vi "1基礎題-Enum-combo box.vi"() -> ()   [LabVIEW 2019]
panel:
  in  "Stop":bool
  out "結果":string
  in  "板材":enum16{"¬üªäªO", "§¨ªO"}(ring)
  in  "色號":string(combo)="フ撤━"
  # "選擇不同的板材時，會出現對應的色號選項供使用者選擇\n並在結果顯示使用者選擇的結果"
  # "Enum"
  # "Combo Box"
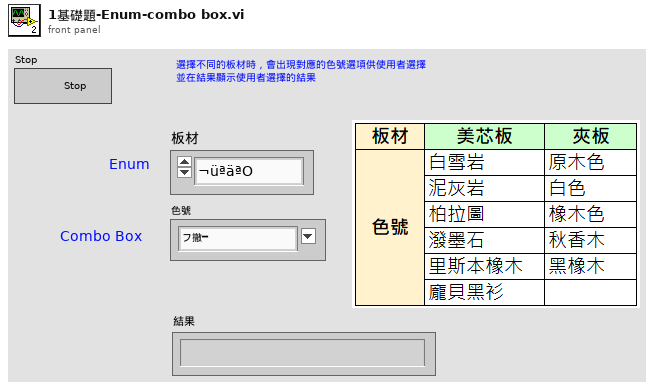
[diagram p1: front panel]
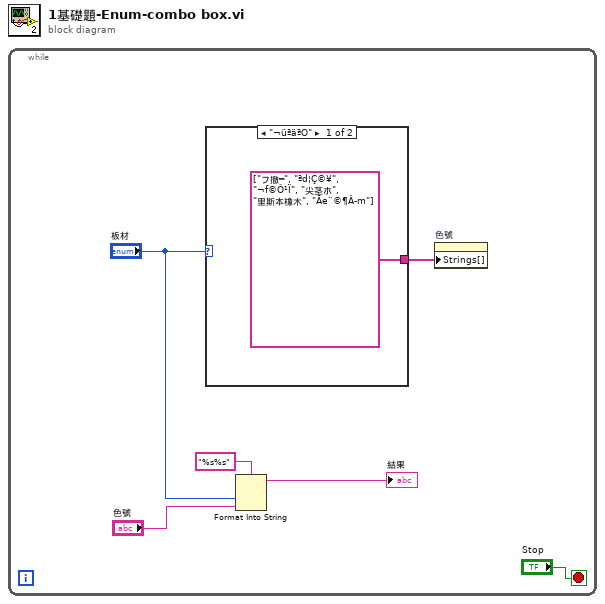
[diagram p0: block diagram]
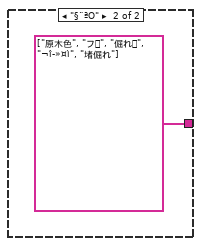
[diagram p2: hidden frame]
diagram:
  n1 = while {
    stop <- "Stop" stop-if-true
    n2 = case shown="\"¬üªäªO\"" "板材" {
      tunnel: [string[] ["フ撤━", "ªd¦Ç©¥", "¬f©Ô¹Ï", "尖茎ホ", "里斯本橡木", "Ãe¨©¶Â­m"] ("Strings []") string[] ["原木色", "フ︹", "倔れ︹", "¬î­»¤ì", "堵倔れ"] ("Strings []")] -> w6
      frame "¬üªäªO" {
      }
      frame "§¨ªO" {
      }
    }
    n3 = Format Into String(format string="%s%s", "板材", "色號") -> (resulting string=→"結果":string)  [unwired: 2 in, 1 out]
    n4 = property on="色號" class="CmbBox"("Strings[]"=w6) -> ()  [unwired: 2 in, 2 out]
  }
